vi "Pet Feeder.vi"() -> ()   [LabVIEW 2023]
panel:
  in  "Timer":dbl
  in  "Consume":bool
  out "STORAGE":dbl(knob) scale=0.0..1000.0
  out "BOWL":dbl(knob) scale=0.0..500.0
  out "Need Refill":bool
  out "Current Storage":dbl
  in  "Min Storage":dbl
  in  "Max Storage":dbl
  in  "Consumption":dbl
  in  "Max bowl level":dbl
  out "Current Bowl":dbl
  in  "Min bowl level":dbl
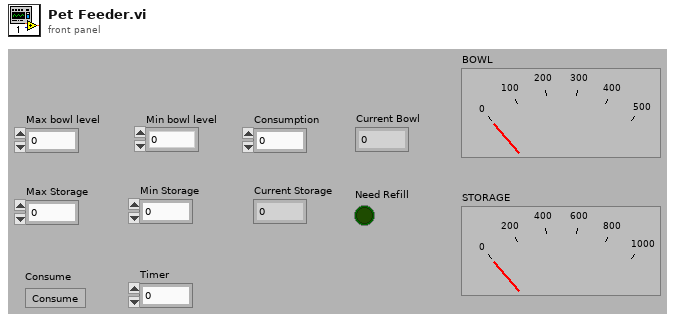
[diagram p1: front panel]
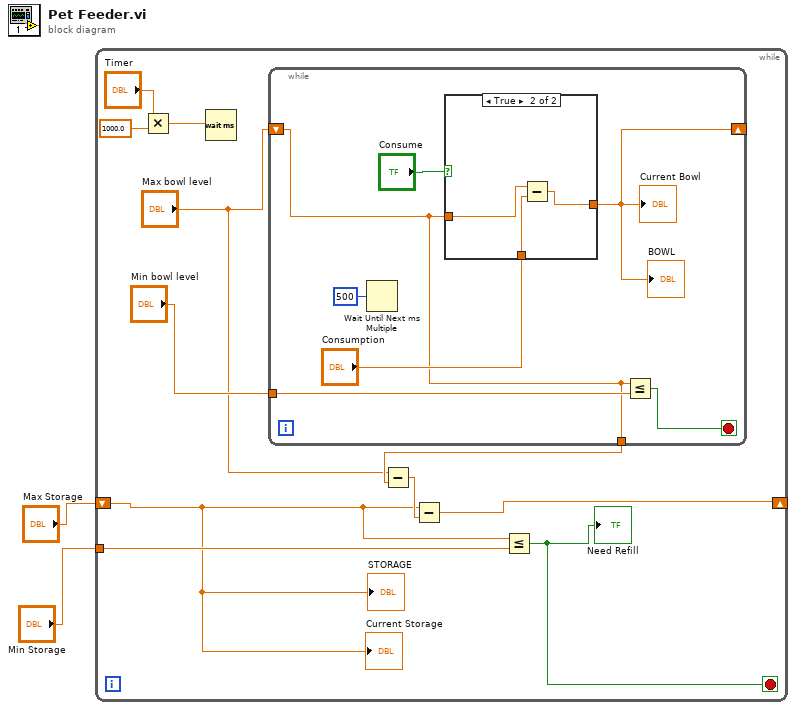
[diagram p0: block diagram]
diagram:
  n1 = while {
    shift-right: [w11] -> _
    shift-left: "Max Storage" -> [w6]
    tunnel: "Min Storage" -> [w10]
    stop <- w9 stop-if-true
    n2 = Multiply(x="Timer", y=1000.0) -> (x*y=w3:dbl)
    n3 = Wait (ms)(milliseconds to wait=w3) -> ()  [unwired: 1 out]
    n4 = while {
      tunnel: [w14] -> w13
      tunnel: "Min bowl level" -> [w19]
      shift-right: [w18] -> _
      shift-left: "Max bowl level" -> [w14]
      stop <- w20 stop-if-true
      n5 = Wait Until Next ms Multiple(millisecond multiple=u32 500) -> ()  [unwired: 1 out]
      n6 = case shown="True" "Consume" {
        tunnel: w14 -> [w21 w24]
        tunnel: "Consumption" -> [_ w23]
        tunnel: [w21 w22] -> w18
        frame False {
        }
        frame True {
          n7 = Subtract(x=w24, y=w23) -> (x-y=w22:dbl)
        }
      }
      "Current Bowl" <- w18
      "BOWL" <- w18
      n8 = Less Or Equal?(x=w14, y=w19) -> (x <= y?=w20:bool)
    }
    n9 = Subtract(x="Max bowl level", y=w13) -> (x-y=w12:dbl)
    n10 = Subtract(x=w6, y=w12) -> (x-y=w11:dbl)
    n11 = Less Or Equal?(x=w6, y=w10) -> (x <= y?=w9:bool)
    "Need Refill" <- w9
    "STORAGE" <- w6
    "Current Storage" <- w6
  }
